vi "SetCurrent -32bit.vi"() -> ()   [LabVIEW 2024]
panel:
  in  "Current":dbl min=0.0 max=1e-06
  in  "stop":bool
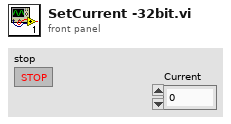
[diagram p1: front panel]
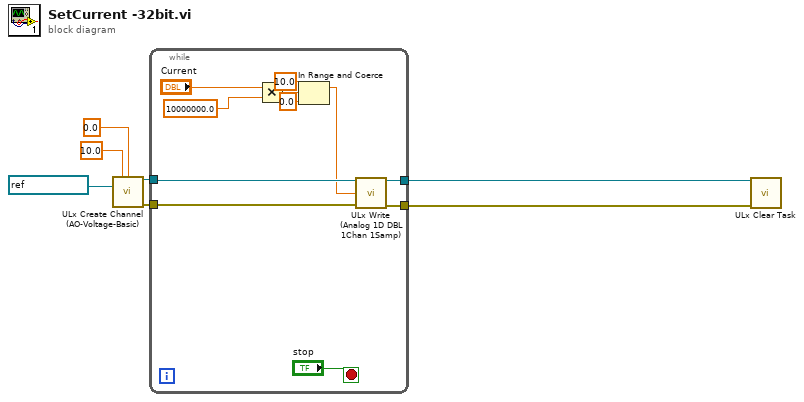
[diagram p0: block diagram]
diagram:
  n1 = call <vilib>:"ULx Create Channel (AO-Voltage-Basic).vi"("maximum value"=10.0, "minimum value"=0.0, "physical channels"=refnum<k21> "Dev0/Ao3") -> ("task out"=w3:refnum<k24>, "error out"=w4:errorcluster)  [unwired: 11 in]
  n2 = while {
    tunnel: w4 -> [w18]
    tunnel: w3 -> [w17]
    tunnel: [w15] -> w2
    tunnel: [w14] -> w1
    stop <- "stop" stop-if-true
    n3 = Multiply(x="Current", y=10000000.0) -> (x*y=w11:dbl)
    n4 = In Range and Coerce(upper limit=10.0, x=w11, lower limit=0.0) -> (coerced(x)=w8:dbl)  [unwired: 1 out]
    n5 = call <vilib>:"ULx Write (Analog 1D DBL 1Chan 1Samp).vi"("task in"=w17, "data"=w8, "error in"=w18) -> ("task out"=w14:refnum<k24>, "error out"=w15:errorcluster)  [unwired: 10 in, 1 out]
  }
  n6 = call <vilib>:"ULx Clear Task.vi"("task in"=w1, "error in"=w2) -> ()  [unwired: 13 in, 1 out]
